vi "Data Sniffer Callback.vi"(7 "Owner":refnum<class>, 10 "Data Direction":T1, 11 "Data":string) -> ()   [LabVIEW 2020, in "Terminal.lvlib" / "Terminal.lvclass"]
uses:
  Terminal.lvclass
  <vilib>/IlluminatedG/lv-stream/stream/Data Direction.ctl
  Terminal.lvclass/Terminal.ctl
  <vilib>/IlluminatedG/lv-stream/Stream.lvlib
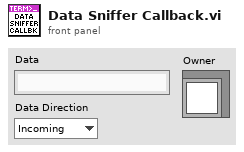
[diagram p1: front panel]
types:
  T1 = typedef "Stream.lvlib/Data Direction.ctl" = enum16{"Incoming", "Outgoing"}
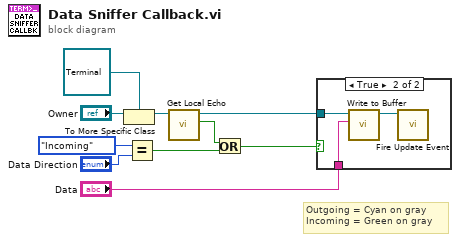
[diagram p0: block diagram]
diagram:
  # "Outgoing = Cyan on gray\nIncoming = Green on gray"
  n1 = To More Specific Class(target class=refnum<class "Terminal.lvclass"> refnum ("Terminal.lvlib:Terminal.lvclass"), reference="Owner") -> (specific class reference=w7:refnum<class "Terminal.lvclass">)  [unwired: 1 in, 1 out]
  n2 = Equal?(x=Data_Direction."Incoming", y="Data Direction") -> (x = y?=w4:bool)
  n3 = call "Get Local Echo.vi"("Terminal in"=w7) -> ("Local Echo"=w3:bool, "Terminal out"=w2:refnum<class "Terminal.lvclass">)  [unwired: 8 in, 1 out]
  n4 = Or(x=w3, y=w4) -> (x .or. y?=w1:bool)
  n5 = case shown="True" w1 {
    tunnel: "Data" -> [_ w13]
    tunnel: w2 -> [_ w12]
    frame False {
    }
    frame True {
      n6 = call "Write to Buffer.vi"("Data"=w13, "Terminal in"=w12) -> ("Terminal out"=w11:refnum<class "Terminal.lvclass">)  [unwired: 8 in, 1 out]
      n7 = call "Fire Update Event.vi"("Terminal in"=w11) -> ()  [unwired: 9 in, 2 out]
    }
  }
